vi "Shooter Controller.vi"(8 "error in":errorcluster) -> ()   [LabVIEW 2015]
doc: "This VI executes continuously carrying out the current operation and responding to updates or new operations. It will often contain the timing or control code that is difficult to place directly in TeleOp. This VI generally opens all sensors and motors and isolates the rest of the robot code from knowing how the operations are carried out."
uses:
  Shooter Setpoints.ctl
  Shooter Operations.ctl
  <vilib>/Rock Robotics/WPI/CAN/TalonSRX/WPI_CANTalonSRX_APIControlMode.ctl
  <vilib>/Rock Robotics/WPI/CAN/TalonSRX/WPI_CANTalonSRX_APIFeedbackSelect.ctl
  <vilib>/Rock Robotics/WPI/CAN/TalonSRX/WPI_CANTalonSRX_BrakeOverride.ctl
  <vilib>/Rock Robotics/WPI/MotorControl/WPI_MotorControlOpenCANTalonSRX.vi
  Shooter Published Globals.vi
  <vilib>/Rock Robotics/Network Tables/NT Write Boolean.vi
panel:
  out "Current\nCmd":string
  # "Tip: It may be helpful to observe inputs and sensor values.\nYou may also want to display tuning or debugging controls."
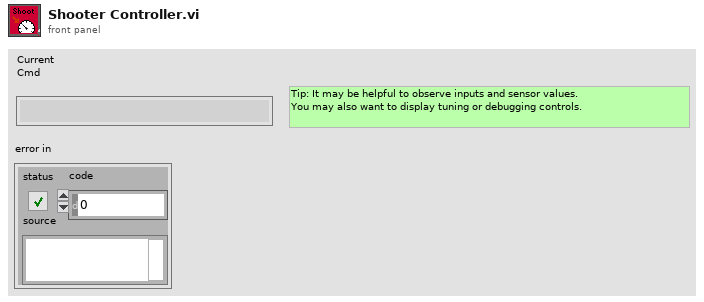
[diagram p1: front panel]
types:
  T1 = typedef "Shooter Setpoints.ctl" = cluster{"Operation":T2, "Setpoint":dbl, "Duration":dbl}
  T2 = typedef "Shooter Operations.ctl" = enum16{"Reserve", "Read Current", "Immediate", "Idle", "Set Speed"}
  T3 = typedef "WPI_CANTalonSRX_BrakeOverride.ctl" = enum8{"No Override", "Override to Coast", "Override to Brake"}
  T4 = typedef "WPI_CANTalonSRX_APIFeedbackSelect.ctl" = enum16{"Digital Quadrature Encoder", "Analog Potentiometer", "Analog Encoder", "Count on Quad-A (Rising-Edge)", "Count on Quad-A (Falling-Edge)", "CTR Magnetic Enc (Absolute)", "CTR Magnetic Enc (Relative)", "Pulse Width"}
  T5 = typedef "WPI_CANTalonSRX_APIControlMode.ctl" = enum8{"Percent VBus", "Speed", "Position", "Slave", "Unchanged / Invalid", "Voltage Compensation", "Current", "Motion Profile"}
  T6 = typedef "WPI_MotorControlDeviceRef.ctl" = cluster{"DeviceStatus":errorcluster, "Type":T7, "PWM":cluster{"PWM Channel":T8, "DeadBand":T9}, "CAN":cluster{"Device Number":u8, "Control Mode":T10, "Semaphore":T11, "Max Vout":dbl, "TalonSRX Control Mode":T5}, "Invert":bool}
  T7 = typedef "WPI_MotorControlType.ctl" = enum16{"PWM", "CAN", "CANTalonSRX"}
  T8 = typedef "FPGA_DIOPWMChannel.ctl" = enum8{"PWM 0", "PWM 1", "PWM 2", "PWM 3", "PWM 4", "PWM 5", "PWM 6", "PWM 7", "PWM 8", "PWM 9", "PWM MXP 0", "PWM MXP 1", "PWM MXP 2", "PWM MXP 3", "PWM MXP 4", "PWM MXP 5", "PWM MXP 6", "PWM MXP 7", "PWM MXP 8", "PWM MXP 9", "Invalid"}
  T9 = typedef "WPI_PWMDeadband.ctl" = cluster{"Name":string, "maxPositivePwm":i32, "minPositivePwm":i32, "centerPwm":i32, "maxNegativePwm":i32, "minNegativePwm":i32, "angularRange":u16}
  T10 = typedef "WPI_CANJaguar_ControlMode.ctl" = enum8{"Percent VBus", "Current", "Speed", "Position", "Voltage"}
  T11 = typedef "Semaphore RefNum" = refnum<k1>
  T12 = typedef "Command Status Info.ctl" = cluster{"Name":string, "Status":T13, "notifier out":T14}
  T13 = typedef "Completion Status.ctl" = enum16{"Successful", "Aborted", "Incomplete"}
  T14 = typedef "Completion Notifier.ctl" = refnum<notifier>
  T15 = cluster{"Default Command":T1, "Command Timing":cluster{"Start Time (ms)":u32, "Iterations":i32}, "Command Arguments":cluster{"Command Info":T12, "Description":string, "Default Command":T1, "notifier out":refnum<notifier>, "Subsystem Name":string}}
  T16 = typedef "WPI_CANTalonSRX_GlobalStatus.ctl" = cluster{"Applied Throttle":dbl, "Module Enabled":bool, "CAN Error":errorcluster, "Closed Loop Error":dbl, "Forward Limit Switch Closed":bool, "Reverse Limit Switch Closed":bool, "Sensor Position":dbl, "Sensor Velocity":dbl, "Current":dbl, "Sticky Fault - Over Temp":bool, "Sticky Fault - Under Voltage":bool, "Sticky Fault - Forward Limit":bool, "Sticky Fault - Reverse Limit":bool, "Sticky Fault - Forward Soft Limit":bool, "Sticky Fault - Reverse Soft Limit":bool, "Brake is Enabled":bool, "Encoder Position":dbl, "Encoder Velocity":dbl, "Encoder Index Count":dbl, "Encoder A Pin State":bool, "Encoder B Pin State":bool, "Encoder Index Pin State":bool, "Analog In":dbl, "Analog In Velocity":dbl, "Temperature (C)":dbl, "Battery Voltage":dbl, "Control 5 Is Supported":bool, "Current Profile Slot Select":dbl, "Pos Div 8":bool, "Vel Div 4":bool, "Pulse Width Position":i32, "Pulse Width Velocity":i32, "Pulse Width Rise To Rise (us)":i32, "Pulse Width Rise To Fall (us)":i32, "Mot Prof Active Is Under Run":bool, "Mot Prof Active Has Under Run":bool, "Mot Prof Active Is Last":bool, "Mot Prof Active Velocity Only":bool, "Mot Prof Active Is Valid":bool, "Mot Prof Buffer Is Full":bool, "Mot Prof Active Profile Slot Select":i32, "Mot Prof NextID":i32, "Mot Prof Count":i32, "Mot Prof Active Velocity":dbl, "Mot Prof Active Position":dbl, "Mot Prof Output Enable":i32}
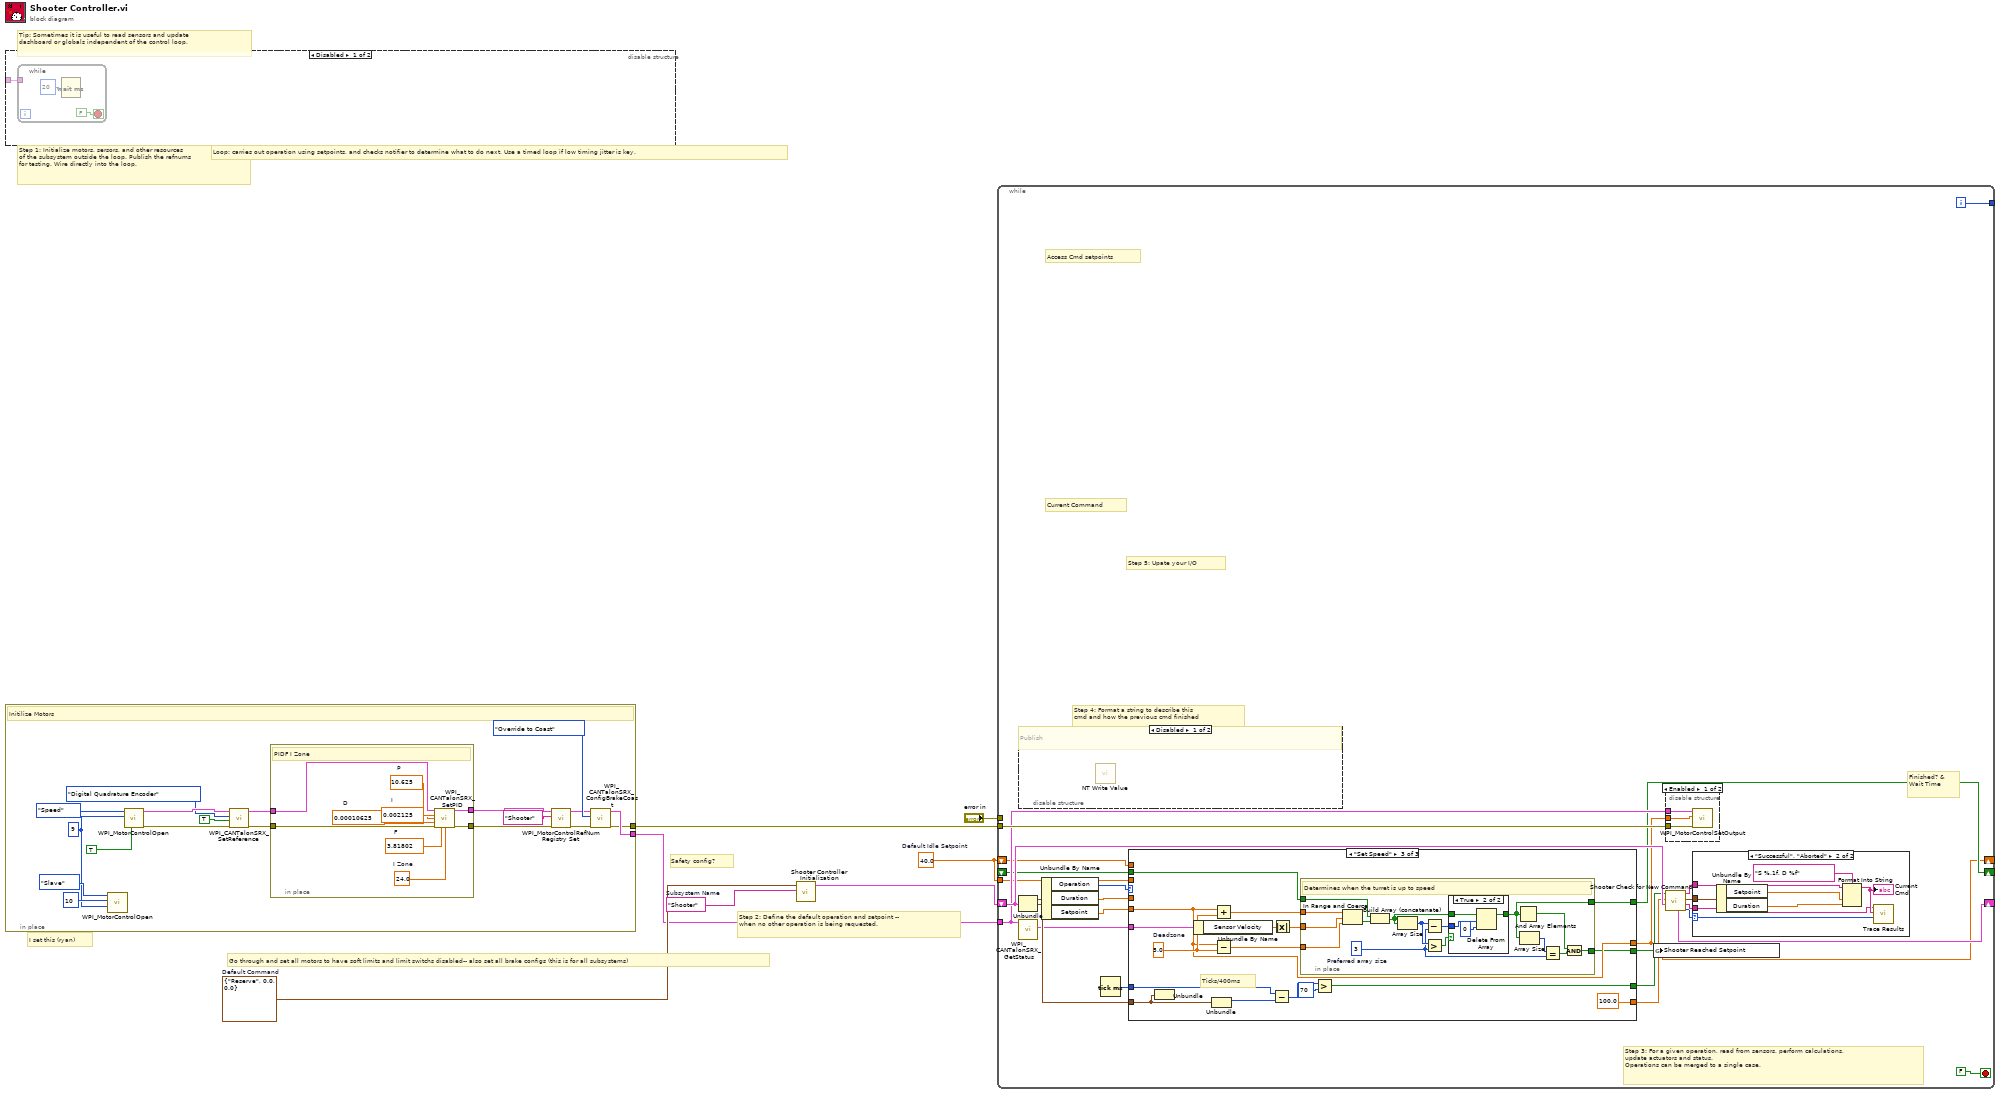
[diagram p0: block diagram]
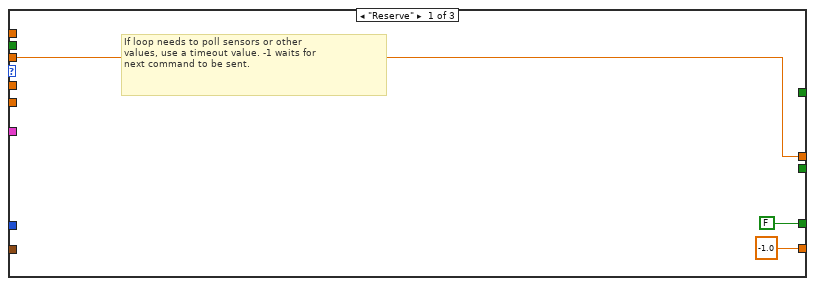
[diagram p6: hidden frame]
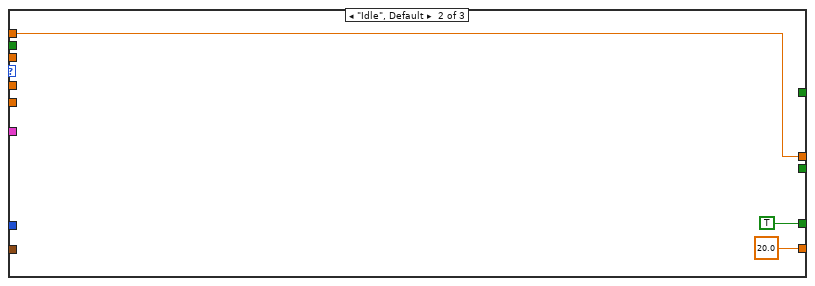
[diagram p7: hidden frame]
diagram:
  w1 = 40.0  # Default Idle Setpoint
  w4 = T1 {"Operation"=enum."Reserve", "Setpoint"=0.0, "Duration"=0.0}  # Default Command
  w5 = "Shooter"  # Subsystem Name
  # "Safety config?"
  # "Go through and set all motors to have soft limits and limit switchs disabled-- also set all brake configs (this is for all subsystems)"
  # "I set this (ryan)"
  # "Tip: Sometimes it is useful to read sensors and update\ndashboard or globals independent of the control loop."
  # "Step 2: Define the default operation and setpoint --\nwhen no other operation is being requested."
  # "Step 1: Initialize motors, sersors, and other resources\nof the subsystem outside the loop. Publish the refnums\nfor testing. Wire directly into the loop."
  # "Loop: carries out operation using setpoints, and checks notifier to determine what to do next. Use a timed loop if low timing jitter is key."
  n1 = disable-structure shown="Disabled" {
    disable-tunnel: _ -> [w8 _]
    frame Disabled {
      n2 = while {
        tunnel: w8 -> [_]
        stop <- FALSE stop-if-true
        n3 = Wait (ms)(milliseconds to wait=u32 20) -> ()  [unwired: 1 out]
      }
    }
    frame Enabled {
    }
  }
  n4 = in-place {
    in-place-border: [w20] -> w3
    in-place-border: [w19] -> w2
    w26 = u8 9 ("Device Number")
    # "Initilize Motors"
    n5 = call-poly <vilib>:"WPI_MotorControlOpen.vi"("Master Device Number"=w26, "Device Number"=u8 10, "Control Mode"=WPI_CANTalonSRX_APIControlMode."Slave") -> ()  [unwired: 7 in, 2 out]
    n6 = call-poly <vilib>:"WPI_MotorControlOpen.vi"("Invert"=TRUE, "Device Number"=w26, "Control Mode"=WPI_CANTalonSRX_APIControlMode."Speed") -> ("error out"=w24:errorcluster, "MotorControlDeviceRef"=w23:T6)  [unwired: 7 in]
    n7 = call <vilib>:"WPI_CANTalonSRX_SetReference.vi"("error in (no error)"=w24, "Reverse Feedback Sensor"=TRUE, "Feedback Reference"=WPI_CANTalonSRX_APIFeedbackSelect."Digital Quadrature Encoder", "CAN Talon SRX Ref"=w23) -> ("error out"=w16:errorcluster, "CAN Talon SRX Ref"=w17:T6)  [unwired: 6 in]
    n8 = in-place {
      in-place-border: [w38] -> w15
      in-place-border: [w37] -> w12
      in-place-border: w17 -> [w36]
      in-place-border: w16 -> [w35]
      w30 = 3.81802  # F
      w31 = 24.0  # I Zone
      w32 = 0.00010625  # D
      w33 = 0.002125  # I
      w34 = 10.625  # P
      # "PIDF I Zone"
      n9 = call <vilib>:"WPI_CANTalonSRX_SetPID.vi"("CAN Talon SRX Ref"=w36, "P"=w34, "I"=w33, "D"=w32, "error in (no error)"=w35, "F"=w30, "I Zone"=w31) -> ("CAN Talon SRX Ref"=w38:T6, "error out"=w37:errorcluster)  [unwired: 7 in]
    }
    n10 = call <vilib>:"WPI_MotorControlRefNum Registry Set.vi"("error in (no error)"=w12, "refnum name"="Shooter", "MotorControlDevRef"=w15) -> ("error out"=w11:errorcluster, "MotorControlDevRef"=w14:T6)  [unwired: 7 in]
    n11 = call <vilib>:"WPI_CANTalonSRX_ConfigBrakeCoast.vi"("error in (no error)"=w11, "Brake / Coast Mode"=WPI_CANTalonSRX_BrakeOverride."Override to Coast", "CAN Talon SRX Ref"=w14) -> ("error out"=w19:errorcluster, "CAN Talon SRX Ref"=w20:T6)  [unwired: 7 in]
  }
  n12 = call "Shooter Controller Initialization.vi"("Subsystem Name"=w5, "Default Command"=w4) -> ("Command Info"=w6:T15)  [unwired: 9 in]
  n13 = while {
    shift-right: [w55] -> _
    shift-left: w6 -> [w56]
    tunnel: [w62] -> _
    tunnel: "error in" -> [_]
    tunnel: w3 -> [w48]
    tunnel: w2 -> [w49]
    shift-right: [w45] -> _
    shift-left: _ -> [w46]
    shift-right: [w44] -> _
    shift-left: w1 -> [w43]
    tunnel: w1 -> [w42]
    i -> [w62]
    stop <- FALSE stop-if-true
    # "Step 5: Upate your I/O"
    # "Step 4: Format a string to describe this\ncmd and how the previous cmd finished"
    # "Current Command"
    # "Access Cmd setpoints"
    # "Finished? &\nWait Time"
    # "Step 3: For a given operation, read from sensors, perform calculations,\nupdate actuators and status.\nOperations can be merged to a single case."
    n14 = disable-structure shown="Disabled" {
      frame Disabled {
        # "Publish"
        n15 = call-poly <vilib>:"NT Write Value.vi"() -> ()  [unwired: 11 in, 1 out]
      }
      frame Enabled {
      }
    }
    n16 = Unbundle(w56) -> ("Default Command"=w61:T1, "Command Timing"=w58:cluster{"Start Time (ms)":u32, "Iterations":i32})  [unwired: 1 out]
    n17 = call <vilib>:"WPI_CANTalonSRX_GetStatus.vi"("CAN Talon SRX Ref"=w48) -> ("Talon SRX Status"=w47:T16)  [unwired: 8 in, 2 out]
    n18 = Unbundle By Name(w61) -> ("Operation"=w40:T2, "Duration"=w60:dbl, "Setpoint"=w57:dbl)
    n19 = Tick Count (ms)() -> (millisecond timer value=w59:u32)
    n20 = case shown="\"Set Speed\"" w40 {
      tunnel: [-1.0 20.0 100.0] -> w54
      tunnel: [FALSE ("ignore previous (F)") TRUE ("ignore previous (F)") w85] -> w39
      tunnel: w58 -> [_ _ w84]
      tunnel: w60 -> [_ _ _]
      tunnel: w59 -> [_ _ w83]
      tunnel: w57 -> [_ _ w93]
      tunnel: [w75 w80 w93] -> w44
      tunnel: w47 -> [_ _ w97]
      tunnel: w46 -> [_ _ w92]
      tunnel: [_ _ w89] -> w45
      tunnel: w43 -> [_ w80 _]
      tunnel: w42 -> [w75 _ _]
      tunnel: [_ _ w82] -> w41
      frame "Reserve" {
        # "If loop needs to poll sensors or other\nvalues, use a timeout value. -1 waits for\nnext command to be sent."
      }
      frame "Idle", Default {
      }
      frame "Set Speed" {
        w94 = 5.0  # Deadzone
        # "Ticks/400ms"
        n21 = Unbundle(w84) -> ()  [unwired: 2 out]
        n22 = Unbundle By Name(w97) -> ("Sensor Velocity"=w90:dbl)
        n23 = Unbundle(w84) -> ("Start Time (ms)"=w86:u32)  [unwired: 1 out]
        n24 = Add(x=w93, y=w94) -> (x+y=w96:dbl)
        n25 = Subtract(x=w93, y=w94) -> (x-y=w95:dbl)
        n26 = Subtract(x=w83, y=w86) -> (x-y=w87:u32)
        n27 = Absolute Value(x=w90) -> (abs(x)=w81:dbl)
        n28 = in-place {
          in-place-border: w96 -> [w112]
          in-place-border: w95 -> [w111]
          in-place-border: w92 -> [w109]
          in-place-border: [w102] -> w89
          in-place-border: [w99] -> w82
          in-place-border: w81 -> [w98]
          w103 = 3  # Preferred array size
          # "Determines when the turret is up to speed"
          n29 = In Range and Coerce(upper limit=w112, x=w98, lower limit=w111) -> (In Range?=w110:bool)  [unwired: 1 out]
          n30 = Build Array (concatenate)(w109, w110) -> (w108:bool[])
          n31 = Array Size(array=w108) -> (size(s)=w106:i32)
          n32 = Subtract(x=w106, y=w103) -> (x-y=w105:i32)
          n33 = Greater?(x=w106, y=w103) -> (0:w107:bool)
          n34 = case shown="True" w107 {
            tunnel: w108 -> [w113 w117]
            tunnel: [w113 w116] -> w102
            tunnel: w105 -> [_ w115]
            frame False {
            }
            frame True {
              n35 = Delete From Array(array=w117, length=w115, index=0) -> (array with subset deleted=w116:bool[])  [unwired: 1 out]
            }
          }
          n36 = And Array Elements(Boolean array=w102) -> (logical AND=w104:bool)
          n37 = Array Size(array=w102) -> (size(s)=w100:i32)
          n38 = Equal?(x=w100, y=w103) -> (x = y?=w101:bool)
          n39 = And(x=w104, y=w101) -> (x .and. y?=w99:bool)
        }
        n40 = Greater?(x=w87, y=u8 70 ("Left Motor")) -> (0:w85:bool)
      }
    }
    n41 = global write "Shooter Published Globals.vi" "Shooter Reached Setpoint"(w41) -> ()
    n42 = disable-structure shown="Enabled" {
      disable-tunnel: w49 -> [w66 _]
      disable-tunnel: w48 -> [w65 _]
      disable-tunnel: w44 -> [w64 _]
      frame Enabled {
        n43 = call <vilib>:"WPI_MotorControlSetOutput.vi"("error in (no error)"=w66, "Output"=w64, "MotorControlDevRef"=w65) -> ()  [unwired: 6 in, 3 out]
      }
      frame Disabled {
      }
    }
    n44 = call "Shooter Check for New Command.vi"("Current Command"=w56, "Wait time (ms)"=w54, "Finished?"=w39) -> ("Completion"=w50:T13, "Subsystem Name"=w51:string, "Current Command"=w52:T1, "Initial Trace String"=w53:string, "NextCommand"=w55:T15)  [unwired: 4 in]
    n45 = case shown="\"Successful\", \"Aborted\"" w50 {
      selector: w50 -> [_ w74]
      tunnel: w53 -> [_ w70]
      tunnel: w52 -> [_ w71]
      tunnel: w51 -> [_ w67]
      frame "Incomplete", Default {
        # "Continuing current command"
      }
      frame "Successful", "Aborted" {
        # "Report and setup for next command"
        n46 = Unbundle By Name(w71) -> ("Setpoint"=w73:dbl, "Duration"=w68:dbl)
        n47 = Format Into String(format string="S %.1f, D %f", initial string=w70, w73, w68) -> (resulting string=w69:string)  [unwired: 1 in, 1 out]
        "Current\nCmd" <- w69
        n48 = call <vilib>:"Trace Results.vi"("Status of previous command"=w74, "Description"=w69, "Subsystem"=w67) -> ()  [unwired: 9 in]
      }
    }
  }
